vi "New Q.vi"(5 "Size":i32=-1, 6 "Make Unique (F)":bool, 7 "Base Name":string, 8 "error in":errorcluster) -> (0 "error out":errorcluster, 3 "Q Ref Out":refnum<queue>)   [LabVIEW 2025, in "Q Wrappers.lvlib"]
uses:
  Q Wrappers.lvlib
  Q Packet.ctl
  <vilib>/numeric/Random Number (Range) U64.vi
  <vilib>/numeric/sub_Random U32.vi
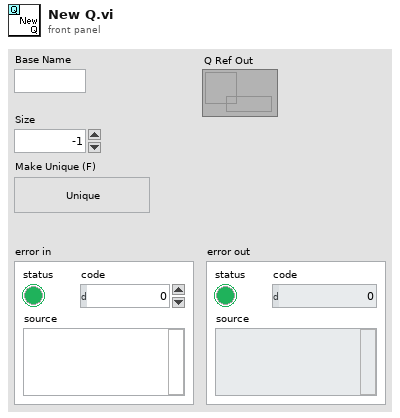
[diagram p1: front panel]
types:
  T1 = typedef "Q Packet.ctl" = cluster{"Packet ID":string, "Payload":variant}
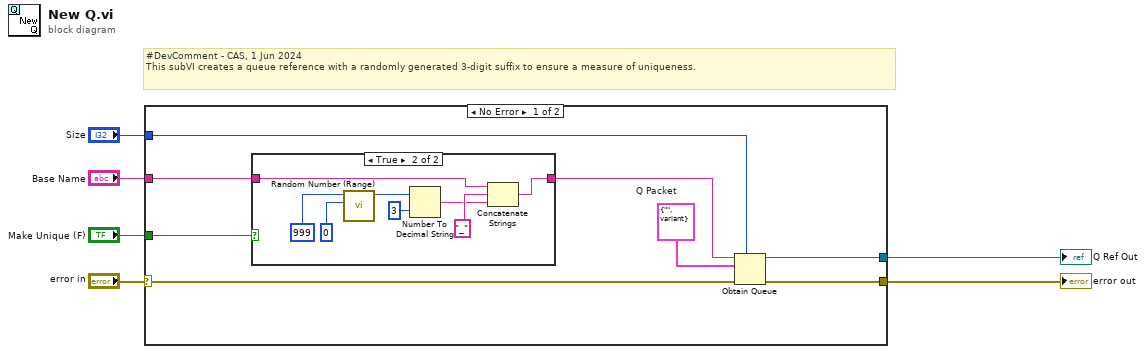
[diagram p0: block diagram]
diagram:
  # "#DevComment - CAS, 1 Jun 2024\nThis subVI creates a queue reference with a randomly generated 3-digit suffix to ensure a measure of uniqueness."
  n1 = case shown="No Error" "error in" {
    selector: "error in" -> [w14 w24]
    tunnel: "Base Name" -> [w9 _]
    tunnel: "Size" -> [w12 _]
    tunnel: [w11 w24] -> w3
    tunnel: [w10 _] -> w2
    tunnel: "Make Unique (F)" -> [w7 _]
    frame No Error {
      w13 = T1 {"Packet ID"="", "Payload"=variant}  # Q Packet
      n2 = case shown="True" w7 {
        tunnel: w9 -> [w15 w23]
        tunnel: [w15 w17] -> w8
        frame False {
        }
        frame True {
          n3 = call-poly <vilib>:"Random Number (Range).vi"("lower bound (0)"=u64 0, "upper bound (100)"=u64 999) -> ("number"=w19:u64)  [unwired: 9 in]
          n4 = Number To Decimal String(number=w19, width (-)=i16 3) -> (decimal integer string=w18:string)
          n5 = Concatenate Strings(w23, "_" ("string"), w18) -> (w17:string)
        }
      }
      n6 = Obtain Queue(max queue size (-1, unlimited)=w12, name (unnamed)=w8, element data type=w13, error in (no error)=w14) -> (queue out=w10:refnum<queue>, error out=w11:errorcluster)  [unwired: 1 in, 1 out]
    }
    frame Error {
    }
  }
  "error out" <- w3
  "Q Ref Out" <- w2
